vi "子VI-缺陷检测界面.vi"(6 "图片/视频路径":path, 7 "图片/视频路径":string, 8 "视频检测帧间隔output":i8, 9 "是否使用GPU计算output":i8, 10 "模式选择output":i8) -> ()   [LabVIEW 2018]
panel:
  out "模型计算时间":string
  out "standard output":string caption="标准输出"
  out "标尺.范围:最大值":dbl
  out "数据库保存路径":path
  out "配置信息说明":string
  out "预测结果保存路径":path
  out "模型预测进度（请等待）":u8(slide) scale=0.0..120.0
  out "模型所在路径":path
  in  "查看结果图-":bool
  out "?":T1(plugin-control)
  out "图片名":string
  out "输出结果文件夹":path caption="路径副本"
  out "预测结果":string
  out "Table":string[][](table) caption="表格"
  in  "表名":string
  in  "数据库选择":bool
  in  "关闭界面":bool
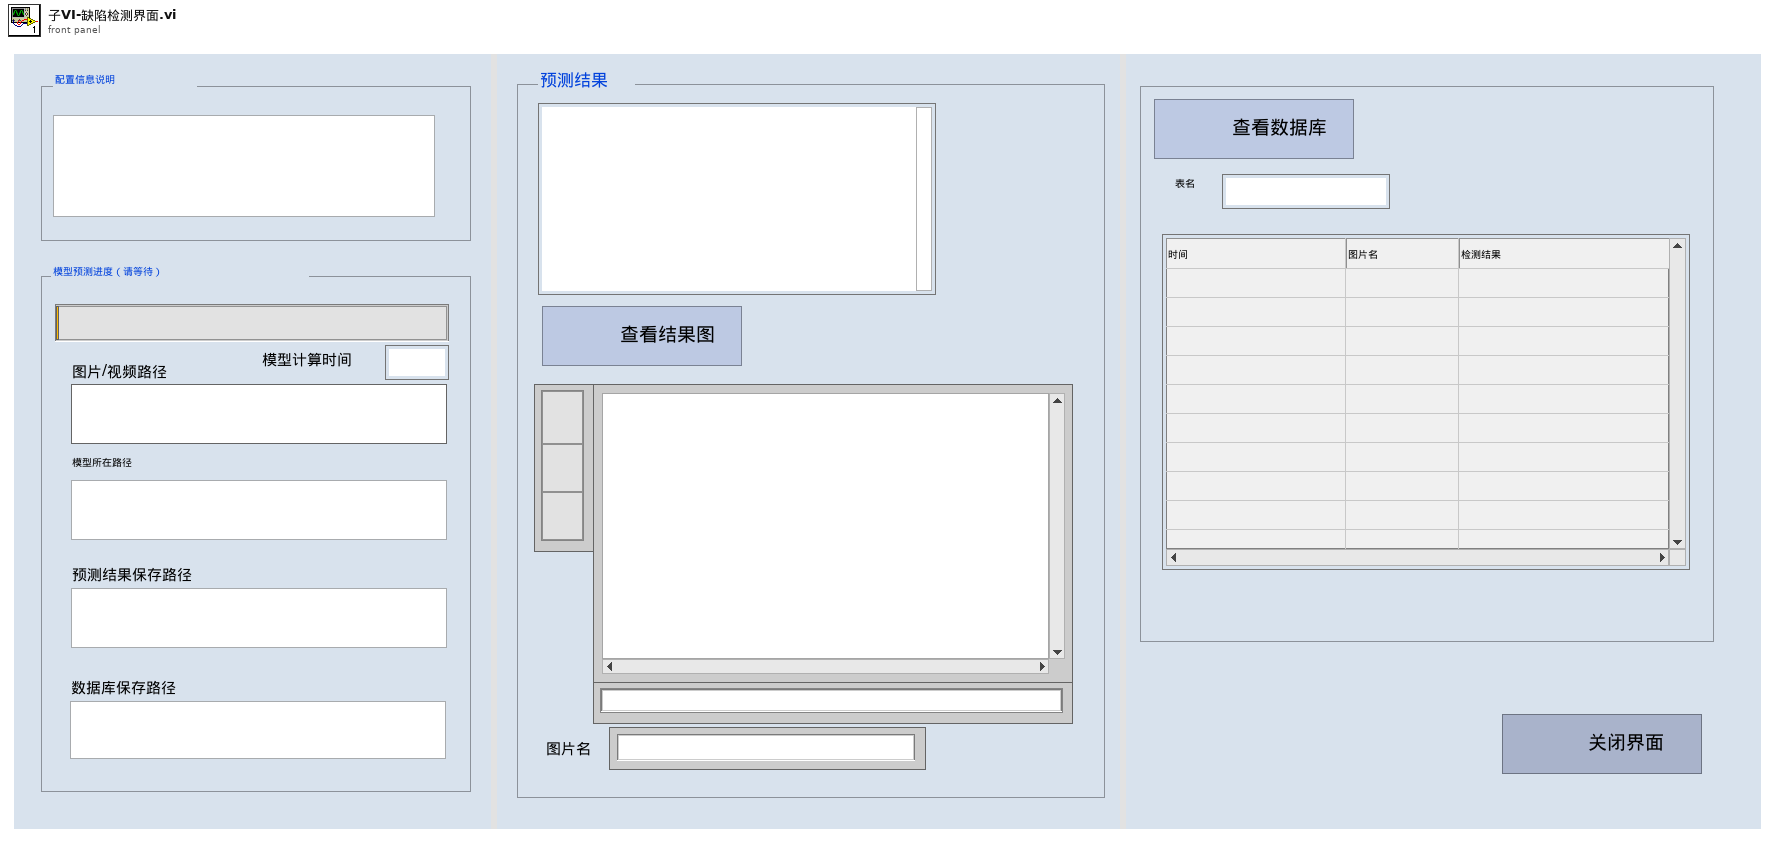
[diagram p1: front panel]
types:
  T1 = typedef "IMAQ Image.ctl" = refnum<image>
  T2 = enum8{"Enabled", "Disabled", "Disabled and Grayed Out"}
  T3 = typedef "Image Type" = u32
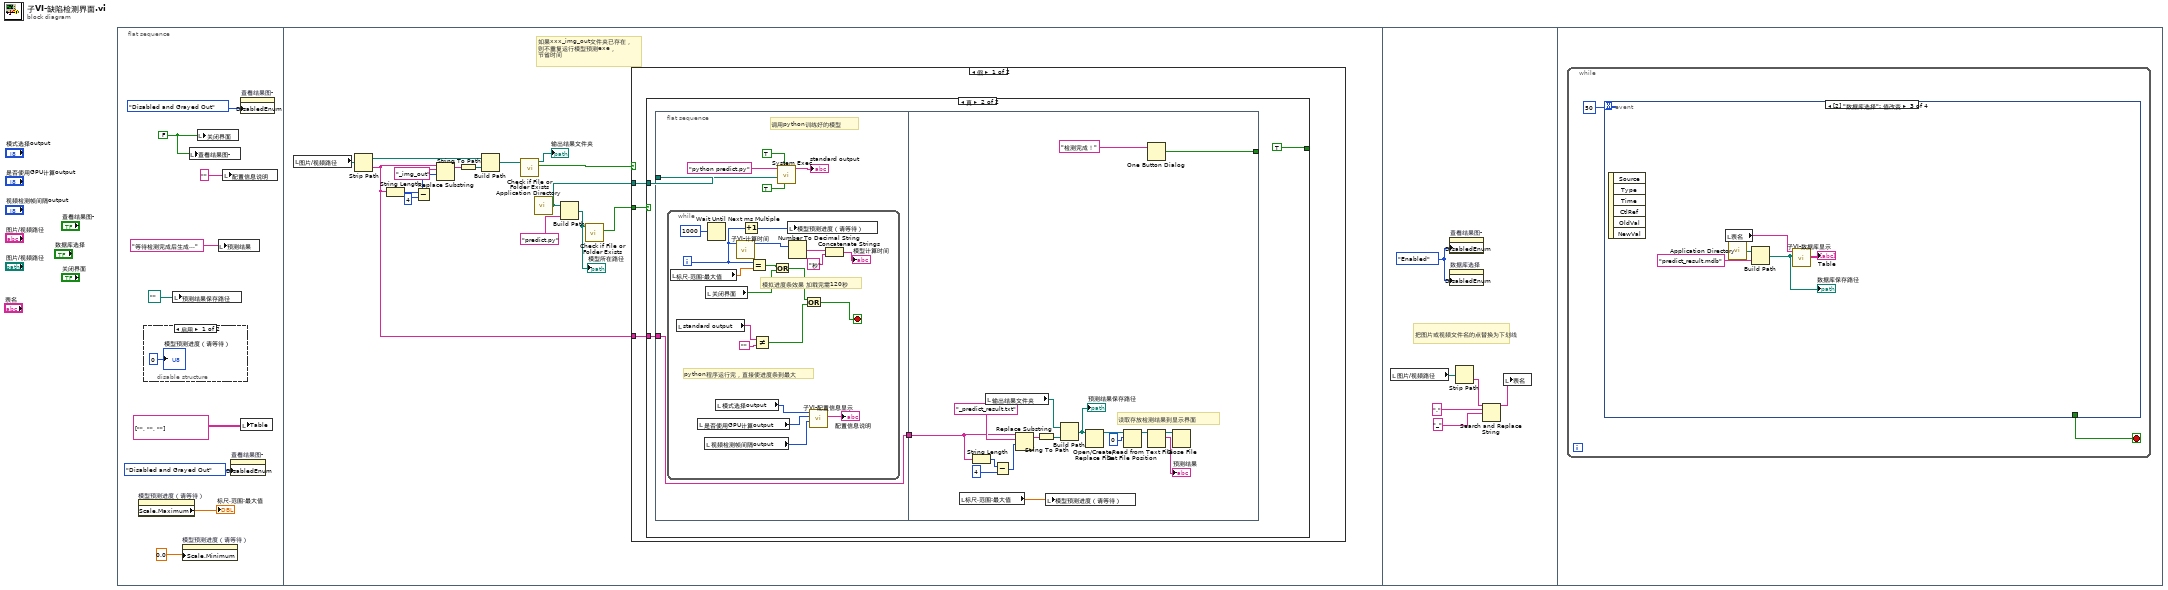
[diagram p0: block diagram]
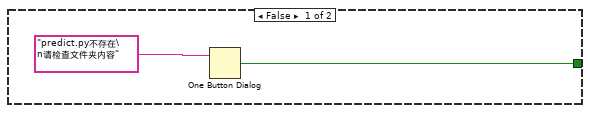
[diagram p3: hidden frame]
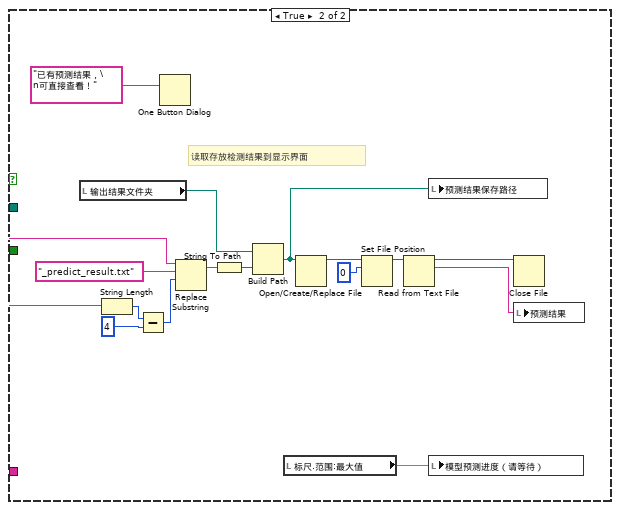
[diagram p4: hidden frame]
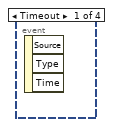
[diagram p5: hidden frame]
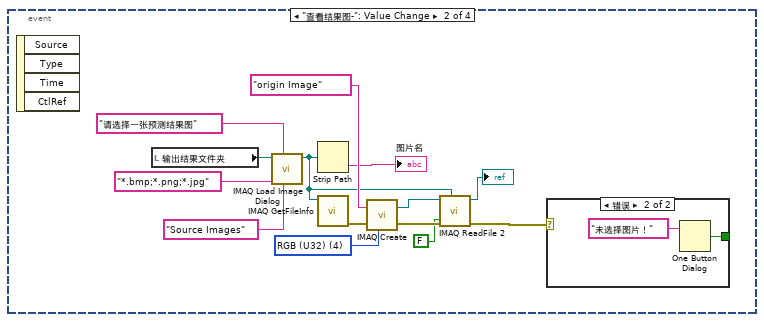
[diagram p6: hidden frame]
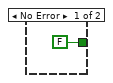
[diagram p7: hidden frame]
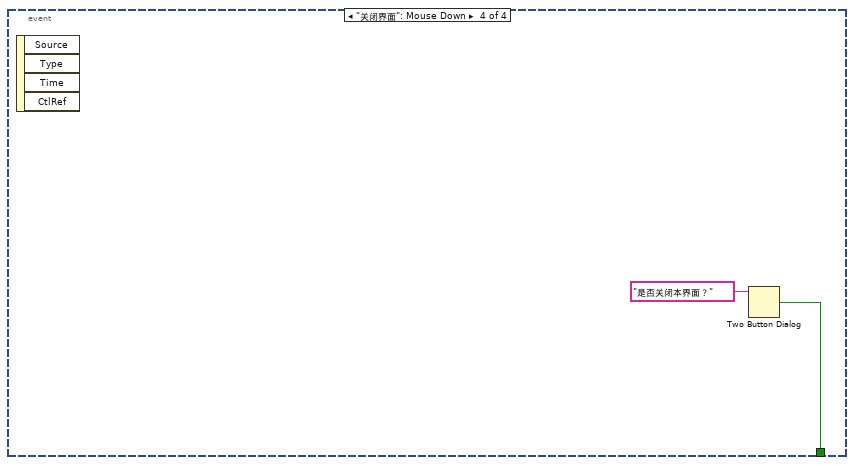
[diagram p8: hidden frame]
diagram:
  n1 = flat-sequence {
    frame #0 {
      w8 = FALSE ("模式选择")
      n2 = property on="模型预测进度（请等待）" class="Slide (严格)"() -> ("Scale.Maximum"=→"标尺.范围:最大值":dbl)  [unwired: 2 in, 2 out]
      n3 = disable-structure shown="启用" {
        frame Enabled {
          "模型预测进度（请等待）" <- u8 0 ("模型运行进度")
        }
        frame Disabled {
        }
      }
      n4 = local write "预测结果保存路径"(path "" ("图片/视频完整路径")) -> ()
      n5 = property on="模型预测进度（请等待）" class="Slide (严格)"("Scale.Minimum"=0.0 ("标尺.范围:最小值")) -> ()  [unwired: 2 in, 2 out]
      n6 = local write "查看结果图-"(w8) -> ()
      n7 = local write "关闭界面"(w8) -> ()
      n8 = local write "预测结果"("等待检测完成后生成...") -> ()
      n9 = local write "配置信息说明"("" ("模式")) -> ()
      n10 = property on="查看结果图-" class="Bool (严格)"("DisabledEnum"=T2."Disabled and Grayed Out" ("禁用")) -> ()  [unwired: 2 in, 2 out]
      n11 = property on="查看结果图-" class="Bool (严格)"("DisabledEnum"=T2."Disabled and Grayed Out" ("禁用")) -> ()  [unwired: 2 in, 2 out]
      n12 = local write "Table"(string[][] [["", "", ""]] ("Table")) -> ()
    }
    frame #1 {
      # "如果xxx_img_out文件夹已存在，\n则不重复运行模型预测exe，\n节省时间"
      n13 = local read "图片/视频路径"() -> (w11:path)
      n14 = Strip Path(path=w11) -> (stripped path=w18:path, name=w23:string)
      n15 = String Length(string=w23) -> (length=w16:i32)
      n16 = Subtract(x=w16, y=4) -> (x-y=w15:i32)
      n17 = Replace Substring(3:w15, 4:"_img_out" ("字符串"), 5:w23) -> (1:w17:string)  [unwired: 1 in, 1 out]
      n18 = String To Path(string=w17) -> (path=w14:path)
      n19 = Build Path(base path=w18, name or relative path=w14) -> (appended path=w25:path)
      n20 = call <vilib>:"Check if File or Folder Exists.vi"("path"=w25) -> ("file or folder exists?"=w26:bool, "dup path"=→"输出结果文件夹":path)  [unwired: 8 in, 1 out]
      n21 = call <vilib>:"Application Directory.vi"() -> ("Application Directory"=w19:path)
      n22 = Build Path(base path=w19, name or relative path="predict.py" ("名称或相对路径")) -> (appended path=w21:path)
      "模型所在路径" <- w21
      n23 = call <vilib>:"Check if File or Folder Exists.vi"("path"=w21) -> ("file or folder exists?"=w20:bool)  [unwired: 8 in, 2 out]
      n24 = case shown="假" w26 {
        tunnel: w23 -> [w29 w83]
        tunnel: w19 -> [w28 _]
        tunnel: w20 -> [w27 _]
        frame False {
          n25 = case shown="真" w27 {
            tunnel: w28 -> [_ w35]
            tunnel: [w31 TRUE ("true")] -> _
            tunnel: w29 -> [_ w32]
            frame False {
              n26 = One Button Dialog(message="predict.py不存在\n请检查文件夹内容" ("消息")) -> (true=w31:bool)  [unwired: 1 in]
            }
            frame True {
              n27 = flat-sequence {
                tunnel: w35 -> [w39]
                tunnel: [w38] -> w33
                tunnel: w32 -> [w38]
                tunnel: w33 -> [w65]
                tunnel: [w63] -> _
                frame #0 {
                  # "调用python训练好的模型"
                  n28 = while {
                    i -> [w47]
                    stop <- w51 stop-if-true
                    # "python程序运行完，直接使进度条到最大"
                    # "模拟进度条效果 加载完需120秒"
                    n29 = local read "标尺.范围:最大值"() -> (w56:dbl)
                    n30 = local read "standard output"() -> (w54:string)
                    n31 = local read "是否使用GPU计算output"() -> (w43:i8)
                    n32 = local read "视频检测帧间隔output"() -> (w42:i8)
                    n33 = local read "关闭界面"() -> (w58:bool)
                    n34 = Wait Until Next ms Multiple(millisecond multiple=u32 1000 ("毫秒倍数")) -> ()  [unwired: 1 out]
                    n35 = local read "模式选择output"() -> (w44:i8)
                    n36 = call "子VI-计算时间.vi"("计算时间"=w47) -> ("计算时间 2"=w46:i32)  [unwired: 10 in]
                    n37 = Increment(x=w47) -> (x+1=w59:i32)
                    n38 = Equal?(x=w47, y=w56) -> (x = y?=w57:bool)
                    n39 = Not Equal?(x=w54, y="") -> (x != y?=w52:bool)
                    n40 = Or(x=w57, y=w58) -> (x .or. y?=w53:bool)
                    n41 = local write "模型预测进度（请等待）"(w59) -> ()
                    n42 = Number To Decimal String(number=w46) -> (decimal integer string=w50:string)  [unwired: 1 in]
                    n43 = Or(x=w53, y=w52) -> (x .or. y?=w51:bool)
                    n44 = call "子VI-配置信息显示.vi"("视频检测帧间隔output"=w42, "是否使用GPU计算output"=w43, "模式选择output"=w44) -> ("配置信息说明"=→"配置信息说明":string)  [unwired: 8 in]
                    n45 = Concatenate Strings(w50, "秒" ("字符串")) -> (→"模型计算时间":string)
                  }
                  n46 = call <vilib>:"System Exec.vi"("run minimized? (F)"=TRUE, "wait until completion? (T)"=TRUE, "working directory"=w39, "command line"="python predict.py") -> ("standard output"=→"standard output":string)  [unwired: 4 in, 3 out]
                }
                frame #1 {
                  # "读取存放检测结果到显示界面"
                  n47 = local read "标尺.范围:最大值"() -> (w61:dbl)
                  n48 = String Length(string=w65) -> (length=w76:i32)
                  n49 = local read "输出结果文件夹"() -> (w62:path)
                  n50 = Subtract(x=w76, y=4) -> (x-y=w77:i32)
                  n51 = Replace Substring(3:w77, 4:"_predict_result.txt" ("字符串"), 5:w65) -> (1:w75:string)  [unwired: 1 in, 1 out]
                  n52 = String To Path(string=w75) -> (path=w74:path)
                  n53 = local write "模型预测进度（请等待）"(w61) -> ()
                  n54 = Build Path(base path=w62, name or relative path=w74) -> (appended path=w69:path)
                  "预测结果保存路径" <- w69
                  n55 = Open/Create/Replace File(file path (use dialog)=w69) -> (refnum out=w70:refnum<file>)  [unwired: 5 in, 2 out]
                  n56 = Set File Position(offset (in bytes) (0)=i64 0 ("偏移量（字节）（0）"), refnum=w70) -> (refnum out=w71:refnum<file>)  [unwired: 2 in, 1 out]
                  n57 = One Button Dialog(message="检测完成！" ("消息")) -> (true=w63:bool)  [unwired: 1 in]
                  n58 = Read from Text File(file (use dialog)=w71) -> (refnum out=w73:refnum<file>, text=→"预测结果":string)  [unwired: 3 in, 2 out]
                  n59 = Close File(refnum=w73) -> ()  [unwired: 1 in, 2 out]
                }
              }
            }
          }
        }
        frame True {
          # "读取存放检测结果到显示界面"
          n60 = local read "输出结果文件夹"() -> (w80:path)
          n61 = String Length(string=w83) -> (length=w85:i32)
          n62 = Subtract(x=w85, y=4) -> (x-y=w84:i32)
          n63 = One Button Dialog(message="已有预测结果，\n可直接查看！" ("消息")) -> ()  [unwired: 1 in, 1 out]
          n64 = Replace Substring(3:w84, 4:"_predict_result.txt" ("字符串"), 5:w83) -> (1:w86:string)  [unwired: 1 in, 1 out]
          n65 = String To Path(string=w86) -> (path=w87:path)
          n66 = Build Path(base path=w80, name or relative path=w87) -> (appended path=w82:path)
          n67 = local read "标尺.范围:最大值"() -> (w78:dbl)
          n68 = Open/Create/Replace File(file path (use dialog)=w82) -> (refnum out=w90:refnum<file>)  [unwired: 5 in, 2 out]
          n69 = Set File Position(offset (in bytes) (0)=i64 0 ("偏移量（字节）（0）"), refnum=w90) -> (refnum out=w89:refnum<file>)  [unwired: 2 in, 1 out]
          n70 = Read from Text File(file (use dialog)=w89) -> (refnum out=w88:refnum<file>, text=w81:string)  [unwired: 3 in, 2 out]
          n71 = local write "预测结果保存路径"(w82) -> ()
          n72 = local write "模型预测进度（请等待）"(w78) -> ()
          n73 = Close File(refnum=w88) -> ()  [unwired: 1 in, 2 out]
          n74 = local write "预测结果"(w81) -> ()
        }
      }
    }
    frame #2 {
      w99 = T2."Enabled" ("禁用")
      # "把图片或视频文件名的点替换为下划线"
      n75 = local read "图片/视频路径"() -> (w98:path)
      n76 = property on="查看结果图-" class="Bool (严格)"("DisabledEnum"=w99) -> ()  [unwired: 2 in, 2 out]
      n77 = property on="数据库选择" class="Bool (严格)"("DisabledEnum"=w99) -> ()  [unwired: 2 in, 2 out]
      n78 = Strip Path(path=w98) -> (name=w95:string)  [unwired: 1 out]
      n79 = Search and Replace String(input string=w95, search string="." ("搜索字符串"), replace string="_" ("子字符串(\"\")")) -> (result string=w94:string)  [unwired: 5 in, 3 out]
      n80 = local write "表名"(w94) -> ()
    }
    frame #3 {
      n81 = while {
        stop <- w100 stop-if-true
        n82 = event shown="[2] \"数据库选择\": 值改变" {
          selector: _ -> [_ _ _ _]
          dyn-events: _ -> [_ _ _ _]
          timeout: 50 -> [_ _ _ _]
          tunnel: [_ _ _ w124] -> w100
          event Timeout {
            n83 = event-data() -> ()  [unwired: 1 in, 3 out]
          }
          event "查看结果图-": Value Change {
            w107 = T3 4 items=["Grayscale (U8)", "Grayscale (I16)", "Grayscale (SGL)", "Complex (CSG)", "RGB (U32)", "HSL (U32)", "RGB (U64)", "Grayscale (U16)"] ("Image Type")
            n84 = event-data() -> ()  [unwired: 1 in, 4 out]
            n85 = local read "输出结果文件夹"() -> (w103:path)
            n86 = call "IMAQ Load Image Dialog"("Pattern Label"="Source Images", "Prompt"="请选择一张预测结果图" ("prompt"), "Pattern"="*.bmp;*.png;*.jpg", "Start Path"=w103) -> ("Path"=w105:path)  [unwired: 5 in, 2 out]
            n87 = Strip Path(path=w105) -> (name=→"图片名":string)  [unwired: 1 out]
            n88 = call "IMAQ GetFileInfo"("File Path"=w105) -> ("error out"=w115:errorcluster)  [unwired: 4 in, 6 out]
            n89 = call "IMAQ Create"("Image Name"="origin Image", "Image Type"=w107, "error in (no error)"=w115) -> ("New Image"=w114:T1, "error out"=w113:errorcluster)  [unwired: 2 in]
            n90 = call "IMAQ ReadFile 2"("Use File Path Image Type"=FALSE, "File Path"=w105, "error in (no error)"=w113, "Image"=w114) -> ("error out"=w106:errorcluster, "Image Out"=→"?":T1)  [unwired: 3 in, 3 out]
            n91 = case shown="错误" w106 {
              tunnel: [FALSE ("true") w117] -> _
              frame No Error {
              }
              frame Error {
                n92 = One Button Dialog(message="未选择图片！" ("消息")) -> (true=w117:bool)  [unwired: 1 in]
              }
            }
          }
          event "数据库选择": Value Change {
            n93 = event-data() -> ()  [unwired: 1 in, 6 out]
            n94 = local read "表名"() -> (w123:string)
            n95 = call <vilib>:"Application Directory.vi"() -> ("Application Directory"=w121:path)
            n96 = Build Path(base path=w121, name or relative path="predict_result.mdb" ("名称或相对路径")) -> (appended path=w120:path)
            "数据库保存路径" <- w120
            n97 = call "子VI-数据库显示.vi"("数据库保存路径"=w120, "表名"=w123) -> ("Table"=→"Table":string[][])  [unwired: 9 in]
          }
          event "关闭界面": Mouse Down {
            n98 = event-data() -> ()  [unwired: 1 in, 4 out]
            n99 = Two Button Dialog(message="是否关闭本界面？" ("消息")) -> (T button?=w124:bool)  [unwired: 2 in]
          }
        }
      }
    }
  }
